vi "Pressure_Temp_Record (SubVI).vi"(4 "Delay Time (s)":dbl=1.0, 6 "Rate":dbl, 9 "Save Data":bool, 10 "PT Filepath":path=path "D:/PDE Project/PDE Data/Default Data/PT.tdms", 11 "TC Filepath":path=path "D:/PDE Project/PDE Data/Default Data/TC.tdms") -> ()   [LabVIEW 2016]
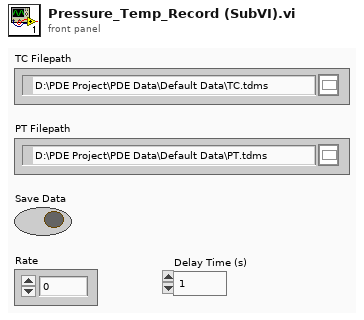
[diagram p1: front panel]
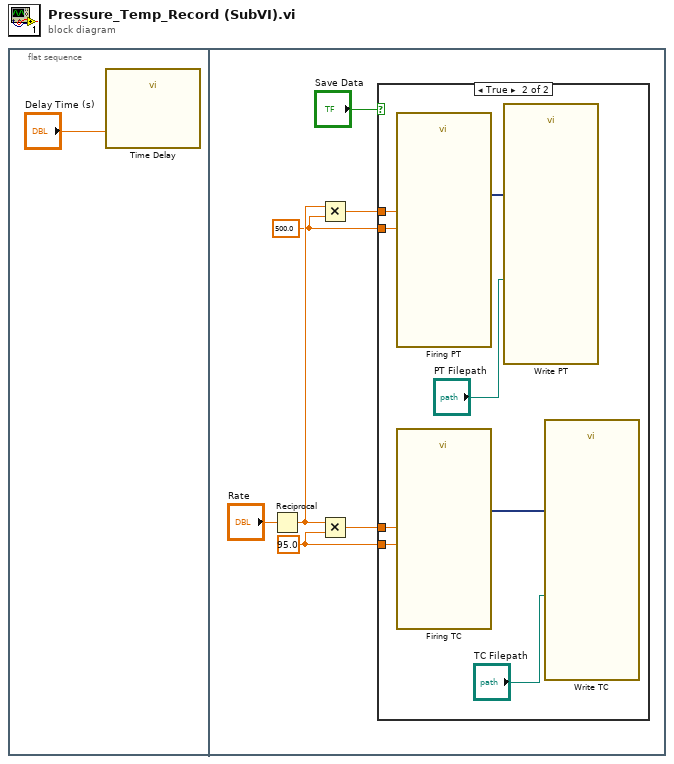
[diagram p0: block diagram]
diagram:
  n1 = flat-sequence {
    frame #0 {
      n2 = call "Time Delay"("Delay Time (s)"="Delay Time (s)") -> ()  [unwired: 10 in, 1 out]
    }
    frame #1 {
      w2 = 95.0 ("rate")
      w4 = 500.0 ("rate")
      n3 = Reciprocal(x="Rate") -> (1/x=w7:dbl)
      n4 = Multiply(x=w7, y=w4) -> (x*y=w5:dbl)
      n5 = Multiply(x=w7, y=w2) -> (x*y=w3:dbl)
      n6 = case shown="True" "Save Data" {
        tunnel: w2 -> [_ w16]
        tunnel: w3 -> [_ w15]
        tunnel: w4 -> [_ w14]
        tunnel: w5 -> [_ w13]
        frame False {
        }
        frame True {
          n7 = call "Firing PT"("rate"=w14, "number of samples"=w13) -> ("data"=w12:dynamicdata)  [unwired: 15 in, 2 out]
          n8 = call "Firing TC"("rate"=w16, "number of samples"=w15) -> ("data"=w11:dynamicdata)  [unwired: 15 in, 2 out]
          n9 = call "Write PT"("Signals"=w12, "Filename"="PT Filepath") -> ()  [unwired: 15 in, 3 out]
          n10 = call "Write TC"("Signals"=w11, "Filename"="TC Filepath") -> ()  [unwired: 15 in, 3 out]
        }
      }
    }
  }
